vi "Global_GearPistonsCTRL.vi"() -> ()   [LabVIEW 2017, in "Gear.lvlib"]
uses:
  Gear.lvlib
  <vilib>/Rock Robotics/WPI/Solenoid/WPI_SolenoidValue.ctl
panel:
  in  "Gear Control":T1
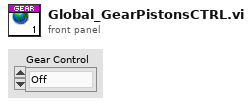
[diagram p1: front panel]
types:
  T1 = typedef "WPI_SolenoidValue.ctl" = enum16{"Off", "On", "Forward", "Reverse"}
diagram:
